vi "WithParent_AddedToParent.vi"() -> (0 "error out":errorcluster)   [LabVIEW 2019, in "ResultTreeTest.lvlib" / "AddTestSuite.lvlib"]
uses:
  2a6c7ef5-d8ea-4de4-ba7d-c6663dbf2225.vi
  Constraint/IsEqual/Create.vi
  Constraint/IsEqual/IsEqual.lvclass
  AddTestSuite.lvlib
  ResultTree/ResultTree.lvclass
panel:
  in  "Tree":string(tree)
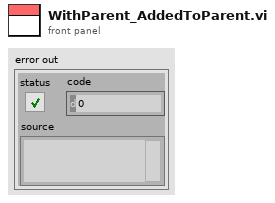
[diagram p1: front panel]
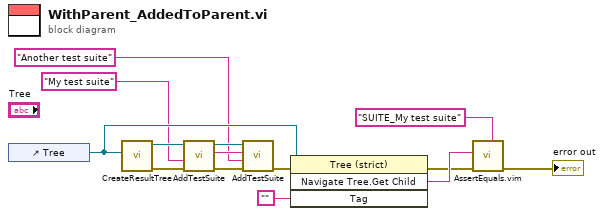
[diagram p0: block diagram]
diagram:
  n1 = control-ref of="Tree"() -> (w13:refnum<vi>)
  n2 = call "CreateResultTree.vi"("Tree Refnum"=w13) -> ("error out"=w12:errorcluster, "ResultTree out"=w11:refnum<class "ResultTree.lvclass">)  [unwired: 9 in]
  n3 = call "AddTestSuite.vi"("error in (no error)"=w12, "Name"="My test suite", "ResultTree in"=w11) -> ("error out"=w5:errorcluster, "Tag Name"=w3:string, "ResultTree out"=w6:refnum<class "ResultTree.lvclass">)  [unwired: 6 in]
  n4 = call "AddTestSuite.vi"("error in (no error)"=w5, "Name"="Another test suite", "Parent Tag (\"\")"=w3, "ResultTree in"=w6) -> ("error out"=w4:errorcluster)  [unwired: 5 in, 2 out]
  n5 = invoke class="Tree (strict)" method="Navigate Tree.Get Child"(reference=w13, error in=w4, "Tag"="") -> (error out=w8:errorcluster, "Navigate Tree:Get Child"=w9:string)  [unwired: 1 in, 2 out]
  n6 = call "AssertEquals.vim"("Expected"="SUITE_My test suite" ("Name"), "error in (no error)"=w8, "Actual"=w9) -> ("error out"=→"error out":errorcluster)  [unwired: 8 in]
